vi "GenerateCode.vi"(1 "Terms":T1[](array[typedef]), 3 "Diagram":refnum<vi>, 5 "XRef":refnum<vi>, 6 "State In":T4) -> (0 "Generated Code?":bool, 2 "State Out":T4, 4 "Reply":string[](array[string]))   [LabVIEW 2015, in "Async-And-Forget.xnode"]
doc: "This ability VI is called when it is time to define the execution behavior of your XNode via LabVIEW's scripting API. This VI is only called when you have previously informed LabVIEW that you need to script through a GenerateCode reply. Diagram is a reference to a diagram of a temporary VI. This diagram contains exactly one front panel terminal for each terminal of your XNode. Terms is an array of pairs of Term IDs and terminal references. LabVIEW will copy code scripted into this diagram into your XNode and connect everything to the correct terminals. The front panel terminals that are on this diagram are special in that they can only be on the top level diagram.\n \n Generate Code? is used to tell LabVIEW whether or not you want to copy the scripted diagram over. If there is an error and you wish not to commit the changes, then the old XNode behavior will be left unchanged. If you set Generate Code? to false, then this VI will be called again next time type propagation is run. Otherwise, it will not be called until you indicate that it should be through the reply on another ability VI.\n \n Because the diagram you are scripting into is separate from the VI containing the XNode instance, type propagation and the data manager will run on the temporary VI after each scripting call.\n \n You should not use the Copy scripting method to move code into the temporary VI. This will adversely affect the user's clipboard. You should use the Move scripting method instead.\n\nDefault behavior: None.\n\nThis ability does not provide UI and OS messages are not handled.\n\nSee also: ModifyCode"
uses:
  Async-And-Forget.xnode
  State.ctl
  <vilib>/Utility/miscctls.llb/LVRectTypeDef.ctl
  <vilib>/picture/picture.llb/imagedata.ctl
  <vilib>/XNodeSupport/XNodeTermIDPair.ctl
  <vilib>/XNodeSupport/XNodeTermRef.ctl
  <vilib>/XNodeSupport/XNodeString.ctl
  <vilib>/Erdos Miller/LV-Scripting/LV-Scripting.lvlib
  <vilib>/XNodeSupport/NI_XNodeSupport.lvlib
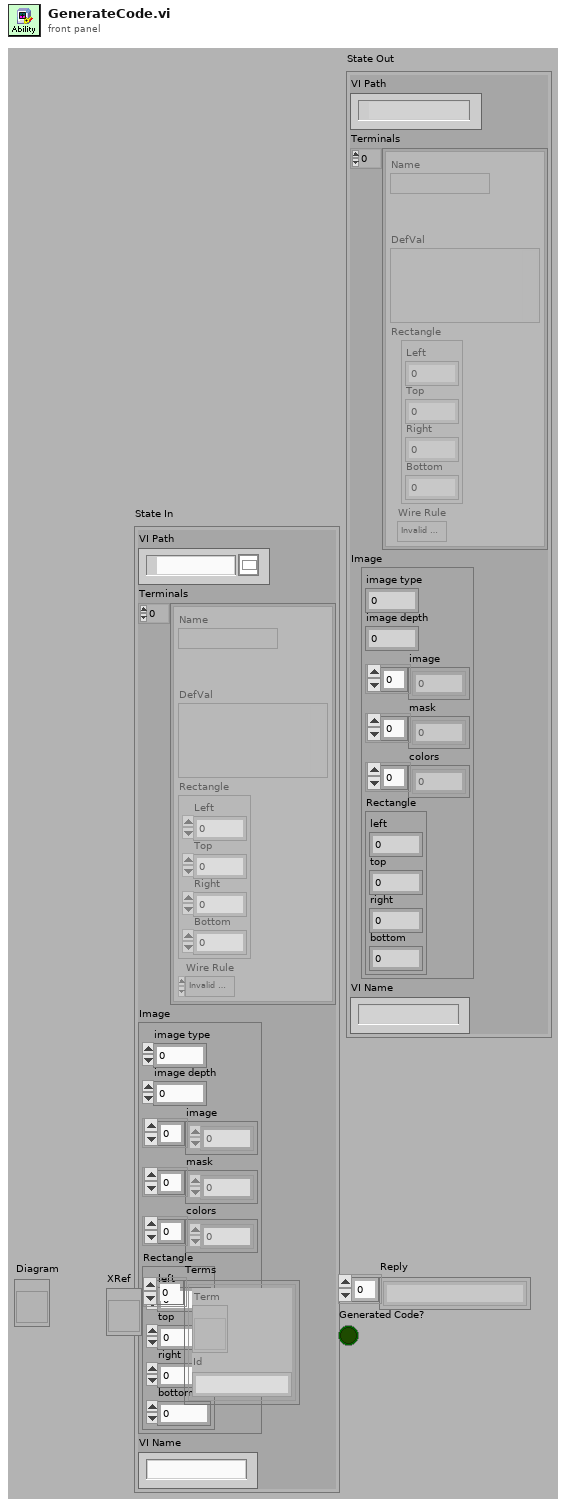
[diagram p1: front panel]
types:
  T1 = typedef "NI_XNodeSupport.lvlib/XNodeTermIDPair.ctl" = cluster{"Term":T2, "Id":T3}
  T2 = typedef "NI_XNodeSupport.lvlib/XNodeTermRef.ctl" = refnum<vi>
  T3 = typedef "NI_XNodeSupport.lvlib/XNodeString.ctl" = string
  T4 = typedef "Async-And-Forget.xnode/State.ctl" = cluster{"VI Path":path, "Terminals":cluster{"Name":string, "DefVal":variant, "Rectangle":T5, "Wire Rule":enum16{"Invalid Wire Rule", "Required", "Recommended", "Optional", "Dynamic Dispatch"}}[], "Image":T6, "VI Name":string}
  T5 = typedef "LVRectTypeDef.ctl" = cluster{"Left":i16, "Top":i16, "Right":i16, "Bottom":i16}
  T6 = typedef "imagedata.ctl" = cluster{"image type":i32, "image depth":i32, "image":u8[], "mask":u8[], "colors":u32[], "Rectangle":cluster{"left":i16, "top":i16, "right":i16, "bottom":i16}}
  T7 = cluster{"Name":string, "DefVal":variant, "Rectangle":T5, "Wire Rule":enum16{"Invalid Wire Rule", "Required", "Recommended", "Optional", "Dynamic Dispatch"}}[]
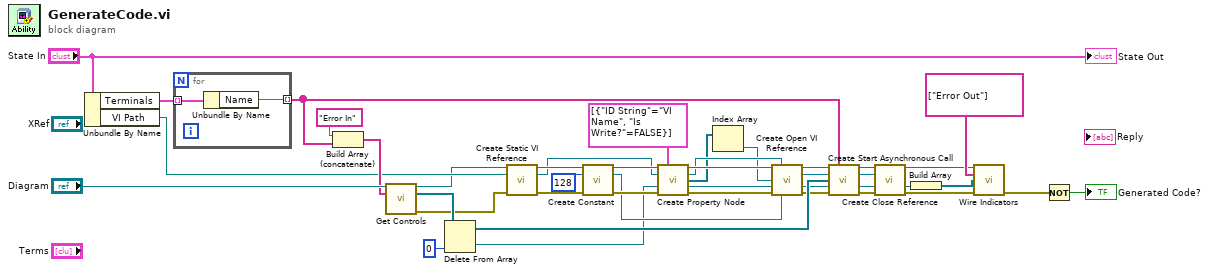
[diagram p0: block diagram]
diagram:
  n1 = Unbundle By Name("State In") -> ("Terminals"=w40:T7, "VI Path"=w35:path)
  n2 = for {
    tunnel: w40 -> [w44] mode=indexing
    tunnel: [w43] -> w24 mode=indexing
    n3 = Unbundle By Name(w44) -> ("Name"=w43:string)
  }
  n4 = Build Array (concatenate)("Error In" ("string"), w24) -> (w38:string[])
  n5 = call <vilib>:"Get Controls.vi"("Diagram in"="Diagram", "Control Names"=w38) -> ("Diagram out"=w34:refnum<vi>, "Control Terminals"=w37:refnum<vi>[], "error out"=w33:errorcluster)  [unwired: 11 in]
  n6 = Delete From Array(array=w37, index=0) -> (deleted portion=w2:refnum<vi>, array with subset deleted=w25:refnum<vi>[])  [unwired: 1 in]
  n7 = call <vilib>:"Create Static VI Reference.vi"("Diagram in"=w34, "VI Path"=w35, "error in (no error)"=w33) -> ("Diagram out"=w22:refnum<vi>, "Terminal"=w6:refnum<vi>, "error out"=w23:errorcluster)  [unwired: 10 in]
  n8 = call <vilib>:"Create Constant.vi"("Diagram in"=w22, "Type"=128, "error in (no error)"=w23) -> ("Diagram out"=w9:refnum<vi>, "Terminal"=w29:refnum<vi>, "error out"=w30:errorcluster)  [unwired: 10 in]
  n9 = call <vilib>:"Create Property Node.vi"("Diagram in"=w9, "Properties"=cluster{"ID String":string, "Is Write?":bool}[] [{"ID String"="VI Name", "Is Write?"=FALSE}], "reference"=w6, "error in"=w2, "error in (no error)"=w30) -> ("Diagram out"=w8:refnum<vi>, "reference out"=w5:refnum<vi>, "Outputs"=w4:refnum<vi>[], 10:"error out"=w1:refnum<vi>, 15:"error out"=w10:errorcluster)  [unwired: 6 in]
  n10 = Index Array(array=w4) -> (element=w3:refnum<vi>)  [unwired: 1 in]
  n11 = call <vilib>:"Create Open VI Reference.vi"("Diagram in"=w8, "type specifier"=w5, "vi path"=w3, "error in"=w1, "error in (no error)"=w10, "options"=w29) -> ("Diagram out"=w21:refnum<vi>, "vi reference"=w19:refnum<vi>, 10:"error out"=w18:refnum<vi>, 15:"error out"=w20:errorcluster)  [unwired: 6 in]
  n12 = call <vilib>:"Create Start Asynchronous Call.vi"("Diagram in"=w21, "Input Names"=w24, "reference"=w19, "Inputs"=w25, "error in"=w18, "error in (no error)"=w20) -> ("Diagram out"=w16:refnum<vi>, "reference out"=w14:refnum<vi>, 10:"error out"=w13:refnum<vi>, 15:"error out"=w26:errorcluster)  [unwired: 6 in]
  n13 = call <vilib>:"Create Close Reference.vi"("Diagram in"=w16, "application reference"=w14, "error in"=w13, "error in (no error)"=w26) -> ("Diagram out"=w15:refnum<vi>, 10:"error out"=w12:refnum<vi>, 15:"error out"=w17:errorcluster)  [unwired: 9 in]
  n14 = Build Array(w12) -> (w11:refnum<vi>[])
  n15 = call <vilib>:"Wire Indicators.vi"("Diagram in"=w15, "Indicator Names"=string[] ["Error Out"], "Outputs"=w11, "error in (no error)"=w17) -> ("error out"=w27:errorcluster)  [unwired: 10 in, 1 out]
  n16 = Not(x=w27) -> (.not. x?=→"Generated Code?":bool)
  "State Out" <- "State In"
